vi "Ctx Shutdown.vi"(7 "path override":path, 8 "error in (no error)":errorcluster, 11 "context_":u32) -> (0 "error out":errorcluster, 3 "context_ out":u32)   [LabVIEW 2025, in "LibZMQ.lvlib"]
doc: "ZMQ_EXPORT int zmq_ctx_shutdown (void *context_);\n\nRelease any blocking calls but doesn't free the context"
uses:
  LibZMQ.lvlib
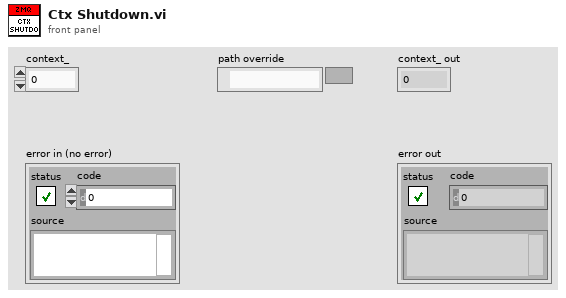
[diagram p1: front panel]
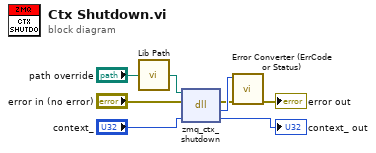
[diagram p0: block diagram]
diagram:
  n1 = call "Lib Path.vi"("path override"="path override") -> ("lib path"=w1:path)
  n2 = dll-call lib="C:/git/ZA/libzmq-v143-mt-4_3_6/lib/win32/libzmq-v143-mt-4_3_6.*" fn="zmq_ctx_shutdown"(path in=w1, error in="error in (no error)", "context_"="context_") -> (error out=w4:errorcluster, "return type"=w8:i32, "context_"=→"context_ out":u32)  [unwired: 1 in, 1 out]
  n3 = call "Error Converter (ErrCode or Status).vi"("error in (no error)"=w4, "error code"=w8) -> ("error out"=→"error out":errorcluster)  [unwired: 9 in]
